vi "FUG-HCN.ProcPeriodic.vi"(0 "i ref in":refnum<vi>, 3 "ms timeout (100)":i32=100, 5 "error in (no error)":errorcluster) -> (14 "i ref out":refnum<vi>, 17 "timed out":bool, 19 "error out":errorcluster)   [LabVIEW 2014, in "FUG-HCN.lvlib"]
doc: "This method serves to periodically do things like reading values from the HW. Methods that should be executed periodically should be called from THIS methode. Add code here."
uses:
  FUG-HCN.lvlib
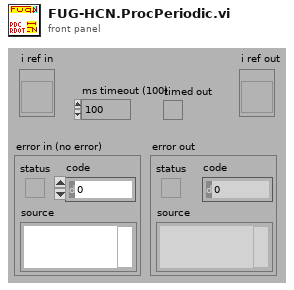
[diagram p1: front panel]
types:
  T1 = typedef "FUG-HCN.lvlib/FUG-HCN.i attribute.ctl" = cluster{"SetStatus":bool, "Set Voltage":dbl, "Nom Voltage":dbl, "VoltageID":i32, "CurrentID":i32}
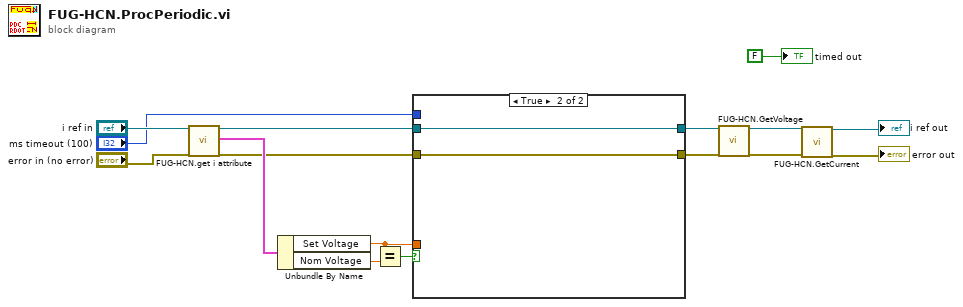
[diagram p0: block diagram]
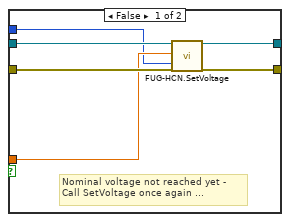
[diagram p2: hidden frame]
diagram:
  n1 = call "FUG-HCN.get i attribute.vi"("i ref in"="i ref in", "error in (no error)"="error in (no error)") -> ("i ref out"=w7:refnum<vi>, "i attribute"=w16:T1, "error out"=w6:errorcluster)  [unwired: 15 in]
  n2 = Unbundle By Name(w16) -> ("Set Voltage"=w8:dbl, "Nom Voltage"=w5:dbl)
  n3 = Equal?(x=w8, y=w5) -> (x = y?=w9:bool)
  n4 = case shown="True" w9 {
    tunnel: w7 -> [w22 w24]
    tunnel: [w18 w24] -> w13
    tunnel: [w17 w23] -> w12
    tunnel: w6 -> [w21 w23]
    tunnel: w8 -> [w20 _]
    tunnel: "ms timeout (100)" -> [w19 _]
    frame False {
      # "Nominal voltage not reached yet - \nCall SetVoltage once again ..."
      n5 = call "FUG-HCN.SetVoltage.vi"("i ref in"=w22, "Set Voltage"=w20, "Time out"=w19, "error in (no error)"=w21) -> ("i ref out"=w18:refnum<vi>, "error out"=w17:errorcluster)  [unwired: 13 in, 1 out]
    }
    frame True {
      # "Nominal Voltage reached the voltage to be set - no action"
    }
  }
  n6 = call "FUG-HCN.GetVoltage.vi"("i ref in"=w13, "error in (no error)"=w12) -> ("i ref out"=w4:refnum<vi>, "error out"=w2:errorcluster)  [unwired: 14 in, 2 out]
  n7 = call "FUG-HCN.GetCurrent.vi"("i ref in"=w4, "error in (no error)"=w2) -> ("i ref out"=→"i ref out":refnum<vi>, "error out"=→"error out":errorcluster)  [unwired: 14 in, 2 out]
  "timed out" <- FALSE ("timed out")
